vi "SV TDMS Write Function Info.vi"(0 "tdms file in":refnum<k34>, 1 "function info":T2 {"function type" items=["Signal"=0, "Speed"=3, "Ratio"=6, "Count"=7, "-"=9, "Level"=10, "-"=19, "Octave Spectrum"=20, "-"=29, "FFT Auto Spectrum"=30, "FFT Cross Spectrum"=40, "Frequency Response"=50, "-"=59, "Event"=90, "None"=98]; "function subtype" items=["Unscaled binary"=0, "Scaled voltage"=1, "Scaled engineering units"=2, "-"=10, "Value"=19, "DC"=11, "AC"=12, "RMS^2"=13, "RMS"=14, "Peak"=15, "Peak to peak"=16, "-"=20, "1/1 octave"=21, "1/3 octave"=22, "1/6 octave"=23, "1/12 octave"=24, "1/24 octave"=25, "-"=30, "Density"=31, "Magnitude"=32, "Phase"=33, "Real"=34, "Imaginary"=35, "Complex"=345, "Coherence"=36, "-"=90, "None"=98, "Unknown"=99]; "X-dimension" items=["Time (s)"=0, "Frequency-CB (Hz)"=1, "Frequency-CPB (Hz)"=1248, "Frequency-Arbitrary (Hz)"=2357, "Quefrency (s)"=2, "Revolutions (rev)"=3, "Order"=4, "Speed (RPM)"=11, "Speed (rad/s)"=21, "Critical Band"=31, "Critical Band Rate (Bark)"=32, "None"=98, "Index"=65535]}, 2 "LabVIEW datatype":T1 items=["String: abc"=7, "Boolean: True or False"=8, "Scalar: y"=0, "Array: Y"=1, "Waveform: t0, dt, Y, variant"=2, "Cluster: x0, dx, Y"=3, "Cluster: X, Y"=4, "Waterfall"=5, "Colormap"=6], 5 "group name":string, 7 "channel name":string, 11 "error in (no error)":errorcluster) -> (4 "tdms file out":refnum<k34>, 6 "group name out":string, 8 "channel name out":string, 15 "error out":errorcluster)   [LabVIEW 2017]
uses:
  <vilib>/addons/_NISVFA/_Shared subVIs/Controls/NI Function Info.ctl
  <vilib>/addons/_NISVFA/_Shared subVIs/Controls/NI Function Type.ctl
  <vilib>/addons/_NISVFA/_Shared subVIs/Controls/NI Function SubType.ctl
  <vilib>/addons/_NISVFA/_Shared subVIs/Controls/svc_X-Axis Units.ctl
  <vilib>/addons/_NISVFA/_Shared subVIs/Controls/LV Datatypes.ctl
  <vilib>/addons/_NISVFA/_Shared subVIs/Controls/NI Channel Properties.ctl
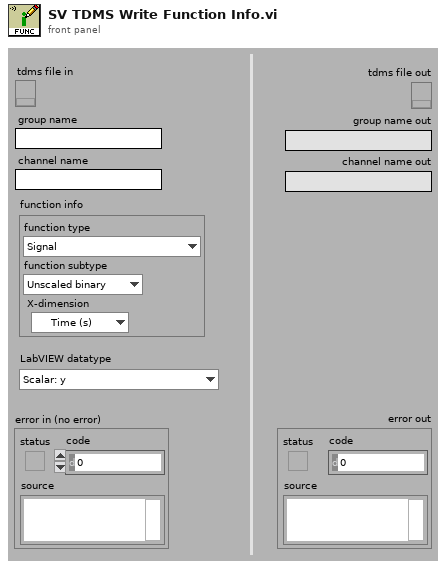
[diagram p1: front panel]
types:
  T1 = typedef "LV Datatypes.ctl" = i32
  T2 = typedef "NI Function Info.ctl" = cluster{"function type":T3, "function subtype":T4, "X-dimension":T5}
  T3 = typedef "NI Function Type.ctl" = u16
  T4 = typedef "NI Function SubType.ctl" = u16
  T5 = typedef "svc_X-Axis Units.ctl" = u16
  T6 = typedef "NI Channel Properties.ctl" = u16
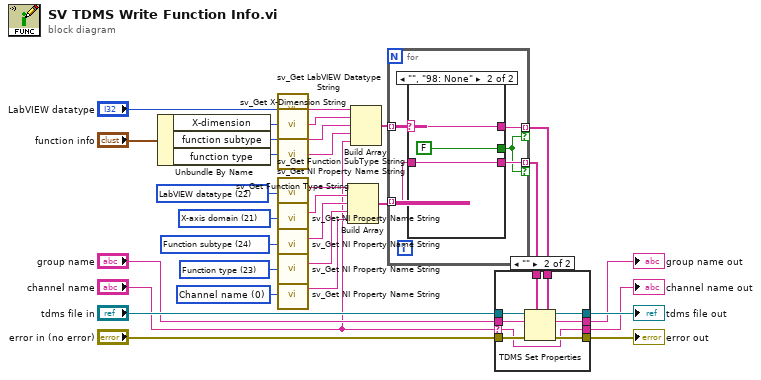
[diagram p0: block diagram]
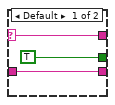
[diagram p2: hidden frame]
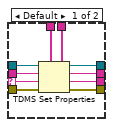
[diagram p3: hidden frame]
diagram:
  w19 = T6 0 items=["Channel name", "Channel description", "Axis label", "Unit string", "Waveform X-axis label", "Waveform X-axis unit string", "x0", "dx", "Number of samples", "X channel", "Filter settled", "dB reference", "Window", "Window parameter", "Window size", "FFT size", "Peak units", "Spectrum type", "Magnitude scale", "Spectral density", "Sensor sensitivity (mV/EU)", "X-axis dimension", "LabVIEW datatype", "Function type", "Function subtype", "X values", "Independent channel"] ("property")
  w20 = T6 22 items=["Channel name", "Channel description", "Y-axis label", "Y-axis unit string", "X-axis label", "X-axis unit string", "x0", "dx", "Number of samples", "X channel", "Filter settled", "dB reference", "Window", "Window parameter", "Window size", "FFT size", "Peak units", "Spectrum type", "Magnitude scale", "Spectral density", "Sensor sensitivity (mV/EU)", "X-axis domain", "LabVIEW datatype"] ("property")
  w25 = T6 24 items=["Channel name", "Channel description", "Y-axis label", "Y-axis unit string", "X-axis label", "X-axis unit string", "x0", "dx", "Number of samples", "X channel", "Filter settled", "dB reference", "Window", "Window parameter", "Window size", "FFT size", "Peak units", "Spectrum type", "Magnitude scale", "Spectral density", "Sensor sensitivity (mV/EU)", "X-axis dimension", "LabVIEW datatype", "Function type", "Function subtype"] ("property")
  w26 = T6 21 items=["Channel name", "Channel description", "Y-axis label", "Y-axis unit string", "X-axis label", "X-axis unit string", "x0", "dx", "Number of samples", "X channel", "Filter settled", "dB reference", "Window", "Window parameter", "Window size", "FFT size", "Peak units", "Spectrum type", "Magnitude scale", "Spectral density", "Sensor sensitivity (mV/EU)", "X-axis domain", "LabVIEW datatype", "Function type", "Component", "Level detector"] ("property")
  w24 = T6 23 items=["Channel name", "Channel description", "Y-axis label", "Y-axis unit string", "X-axis label", "X-axis unit string", "x0", "dx", "Number of samples", "X channel", "Filter settled", "dB reference", "Window", "Window parameter", "Window size", "FFT size", "Peak units", "Spectrum type", "Magnitude scale", "Spectral density", "Sensor sensitivity (mV/EU)", "X-axis domain", "LabVIEW datatype", "Function type", "Component", "Level detector"] ("property")
  n1 = Unbundle By Name("function info") -> ("X-dimension"=w28:T5, "function subtype"=w27:T4, "function type"=w29:T3)
  n2 = call <vilib>:"sv_Get LabVIEW Datatype String.vi"("LabVIEW datatype"="LabVIEW datatype") -> ("datatype string"=w16:string)  [unwired: 4 in]
  n3 = call <vilib>:"sv_Get X-Dimension String.vi"("x-axis units"=w28) -> ("x-domain string"=w15:string)  [unwired: 4 in]
  n4 = call <vilib>:"sv_Get Function SubType String.vi"("function subtype"=w27) -> ("function type string"=w14:string)  [unwired: 4 in]
  n5 = call <vilib>:"sv_Get Function Type String.vi"("function type"=w29) -> ("function type string"=w13:string)  [unwired: 4 in]
  n6 = call <vilib>:"sv_Get NI Property Name String.vi"("property"=w20) -> ("TDMS property name"=w11:string)  [unwired: 13 in, 1 out]
  n7 = call <vilib>:"sv_Get NI Property Name String.vi"("property"=w26) -> ("TDMS property name"=w10:string)  [unwired: 13 in, 1 out]
  n8 = call <vilib>:"sv_Get NI Property Name String.vi"("property"=w25) -> ("TDMS property name"=w9:string)  [unwired: 13 in, 1 out]
  n9 = call <vilib>:"sv_Get NI Property Name String.vi"("property"=w24) -> ("TDMS property name"=w8:string)  [unwired: 13 in, 1 out]
  n10 = call <vilib>:"sv_Get NI Property Name String.vi"("property"=w19) -> ("TDMS property name"=w7:string)  [unwired: 13 in, 1 out]
  n11 = Build Array(w11, w10, w9, w8, w7) -> (w6:string[])
  n12 = Build Array(w16, w15, w14, w13, "channel name") -> (w12:string[])
  n13 = for {
    tunnel: w12 -> [w36] mode=indexing
    tunnel: [w35] -> w5 mode=indexing if=w32
    tunnel: w6 -> [w34] mode=indexing
    tunnel: [w33] -> w4 mode=indexing if=w32
    n14 = case shown="\"\", \"98: None\"" w36 {
      selector: w36 -> [w38 w42]
      tunnel: [w38 w42] -> w35
      tunnel: [TRUE FALSE] -> w32
      tunnel: w34 -> [w37 w40]
      tunnel: [w37 w40] -> w33
      frame Default {
      }
      frame "", "98: None" {
      }
    }
  }
  n15 = case shown="\"\"" "channel name" {
    selector: "channel name" -> [w45 w55]
    tunnel: "tdms file in" -> [w52 w61]
    tunnel: "error in (no error)" -> [w51 w60]
    tunnel: [w50 w59] -> w22
    tunnel: [w49 w58] -> w21
    tunnel: [w48 w57] -> w18
    tunnel: "group name" -> [w47 w56]
    tunnel: [w46 w55] -> w17
    tunnel: w5 -> [w44 w54]
    tunnel: w4 -> [w43 w53]
    frame Default {
      n16 = TDMS Set Properties(5:w44, 7:w43, 8:w51, 9:w45, 10:w47, 11:w52) -> (0:w48:errorcluster, 1:w46:string, 2:w49:string, 3:w50:refnum<k34>)
    }
    frame "" {
      n17 = TDMS Set Properties(5:w54, 7:w53, 8:w60, 10:w56, 11:w61) -> (0:w57:errorcluster, 2:w58:string, 3:w59:refnum<k34>)  [unwired: 1 in, 1 out]
    }
  }
  "error out" <- w18
  "channel name out" <- w17
  "group name out" <- w21
  "tdms file out" <- w22
